vi "New Standard VI.vi"(8 "error in (no error)":errorcluster, 10 "App Refnum":refnum<vi>, 11 "SubVI Refnum":refnum<vi>) -> (0 "error out":errorcluster, 3 "Standard VI Type out":refnum<class "Standard VI Type.lvclass">)   [LabVIEW 2020, in "Peek Window.lvlib" / "Standard VI Type.lvclass"]
uses:
  Standard VI Type.lvclass
  Standard VI Type.lvclass/Standard VI Type.ctl
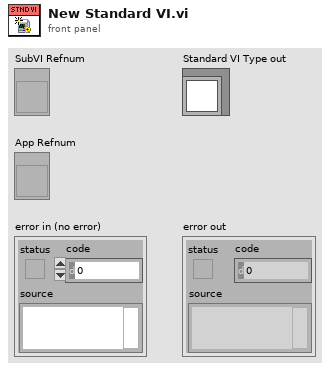
[diagram p1: front panel]
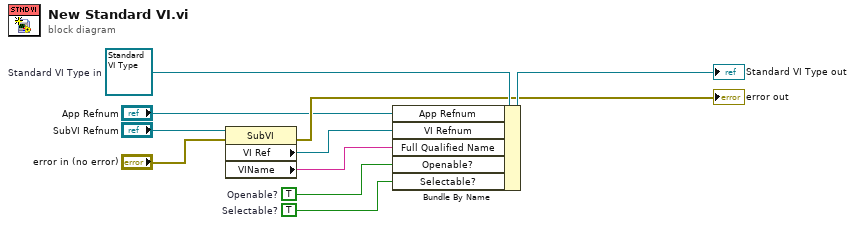
[diagram p0: block diagram]
diagram:
  w1 = TRUE  # Selectable?
  w2 = TRUE  # Openable?
  w10 = refnum<class "Standard VI Type.lvclass"> refnum  # Standard VI Type in
  n1 = property class="SubVI"(reference="SubVI Refnum", error in="error in (no error)") -> (error out=→"error out":errorcluster, "VI Ref"=w3:refnum<vi>, "VIName"=w5:string)  [unwired: 1 out]
  n2 = Bundle By Name(cluster=w10, "App Refnum"="App Refnum", "VI Refnum"=w3, "Full Qualified Name"=w5, "Openable?"=w2, "Selectable?"=w1) -> (→"Standard VI Type out":refnum<class "Standard VI Type.lvclass">)
